vi "Actor Core.vi"(8 "error in":errorcluster, 11 "Laser Process in":refnum<class "Laser Process.lvclass">) -> (0 "error out":errorcluster, 3 "Actor out":refnum<class "Actor.lvclass">)   [LabVIEW 2022 SP3, in "Laser Process.lvlib" / "Laser Process.lvclass"]
doc: "(<B>Filename</B>: Actor Framework.lvlib:Actor.lvclass:Actor Core.vi)\n\nReceives messages to the actor, reacts to them, and initiates any error handling that may shut the actor down.\n\nDescendant classes may override this VI to append parallel tasks for the actor to complete while it handles messages. Overrides use the Call Parent Class Method node."
uses:
  Laser Process.lvclass
  C:/Program Files/National Instruments/LabVIEW 2022/vi.lib/MGI/Monitored Actor/Monitored Actor/Monitored Actor/Monitored Actor.lvclass
  <vilib>/ActorFramework/Actor/Actor.lvclass
  Laser State Data/Time and Temp.ctl
  <vilib>/MGI/Monitored Actor/Monitored Actor/Monitored Actor/Monitored Actor.lvclass/Monitored Actor.ctl
  Laser Process.lvclass/Laser Process.ctl
  Laser State Data/Laser State Data.lvclass/Laser State Data.ctl
  Laser State Data/Write Current Power.vi
  Laser State Data/Write Temp.vi
  Laser State Data/Read Events.vi
  <vilib>/MGI/Monitored Actor/Monitored Actor/Monitored Actor/Monitored Actor.lvclass
  Laser Driver/Laser Driver.lvclass
  Laser State Data/Laser State Data.lvclass
panel:
  out "Time and Temp":T1
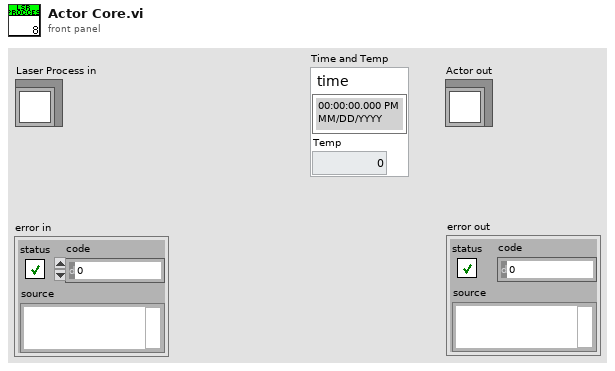
[diagram p1: front panel]
types:
  T1 = typedef "Laser State Data.lvclass/Time and Temp.ctl" = cluster{" time":timestamp, "Temp":dbl}
  T2 = typedef "Laser State Data.lvclass/Events.ctl" = cluster{"Temp":refnum<user-event>, "Current Power":refnum<user-event>, "Laser State":refnum<user-event>, "Time and Temp":refnum<user-event>}
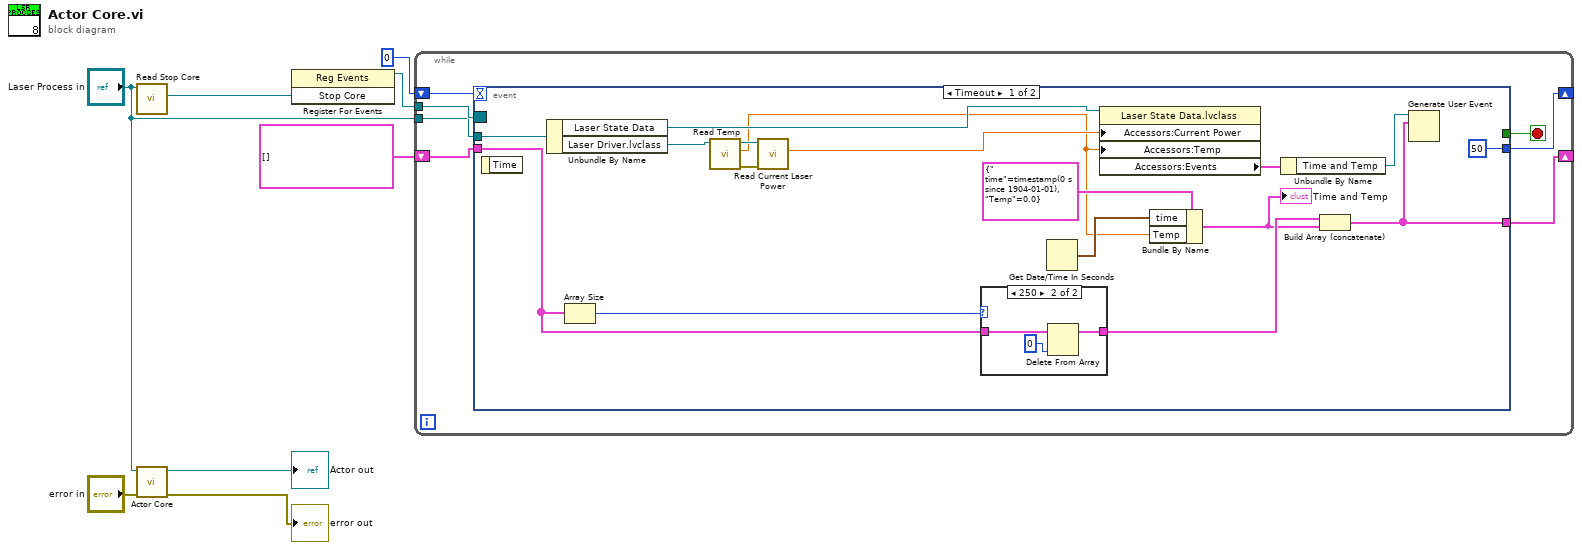
[diagram p0: block diagram]
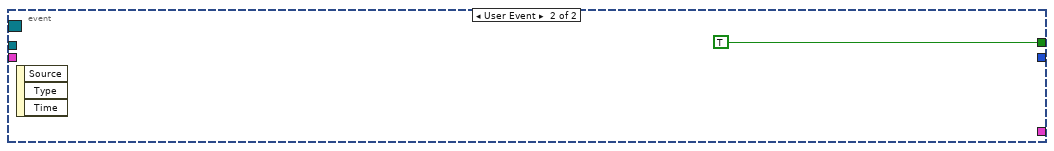
[diagram p3: hidden frame]
diagram:
  n1 = call <vilib>:"Read Stop Core.vi"("Monitored Actor in"="Laser Process in") -> ("Stop Core"=w5:refnum<user-event>)  [unwired: 8 in, 2 out]
  n2 = call-parent "Actor Core.vi"("error in"="error in", "Actor in"="Laser Process in") -> ("error out"=→"error out":errorcluster, "Actor out"=→"Actor out":refnum<class "Actor.lvclass">)  [unwired: 8 in]
  n3 = register-events(w5) -> (reference out=w4:refnum<event-registration>)  [unwired: 2 in, 1 out]
  n4 = while {
    tunnel: w4 -> [w15]
    shift-right: [w12] -> _
    shift-left: 0 -> [w13]
    tunnel: "Laser Process in" -> [w11]
    shift-right: [w10] -> _
    shift-left: T1[] [] -> [w9]
    stop <- w14 stop-if-true
    n5 = event shown="[0] Timeout" {
      selector: w15 -> [_ _]
      dyn-events: _ -> [_ _]
      timeout: w13 -> [_ _]
      tunnel: [_ TRUE] -> w14
      tunnel: [50 _] -> w12
      tunnel: w11 -> [w31 _]
      tunnel: [w18 _] -> w10
      tunnel: w9 -> [w22 _]
      event Timeout {
        n6 = event-data() -> ()  [unwired: 1 in, 1 out]
        n7 = Unbundle By Name(w31) -> ("Laser State Data"=w28:refnum<data-value>, "Laser Driver.lvclass"=w26:refnum<class "Laser Driver.lvclass">)
        n8 = Array Size(array=w22) -> (size(s)=w21:i32)
        n9 = call-dynamic "Read Temp.vi"("Laser Driver in"=w26) -> ("error out"=w30:errorcluster, "Temp"=w23:dbl, "Laser Driver out"=w29:refnum<class "Laser Driver.lvclass">)  [unwired: 8 in]
        n10 = call-dynamic "Read Current Laser Power.vi"("error in (no error)"=w30, "Laser Driver in"=w29) -> ("Current Laser Power"=w27:dbl)  [unwired: 7 in, 2 out]
        n11 = case shown="250" w21 {
          tunnel: w22 -> [w33 w36]
          tunnel: [w33 w34] -> w17
          frame Default {
          }
          frame 250 {
            n12 = Delete From Array(array=w36, index=0) -> (array with subset deleted=w34:T1[])  [unwired: 1 in, 1 out]
          }
        }
        n13 = Get Date/Time In Seconds() -> (seconds since 1Jan1904=w25:timestamp)
        n14 = property class="Laser State Data.lvclass"(reference=w28, "Accessors:Current Power"=w27, "Accessors:Temp"=w23) -> ("Accessors:Events"=w20:T2)  [unwired: 1 in, 2 out]
        n15 = Bundle By Name(cluster=T1 {" time"=timestamp(0 s since 1904-01-01), "Temp"=0.0}, "time"=w25, "Temp"=w23) -> (w16:T1)
        "Time and Temp" <- w16
        n16 = Unbundle By Name(w20) -> ("Time and Temp"=w19:refnum<user-event>)
        n17 = Build Array (concatenate)(w17, w16) -> (w18:T1[])
        n18 = Generate User Event(user event=w19, event data cluster=w18) -> ()  [unwired: 2 in, 2 out]
      }
      event User Event {
        n19 = event-data() -> ()  [unwired: 1 in, 3 out]
      }
    }
  }
